vi "poly_average_ith_value_double.vi"(1 "0 indexed? (T, F = 1 indexed)":bool=TRUE, 2 "new value":dbl format="%#_13g", 3 "old value":dbl=nan format="%#_13g", 4 "i":i32) -> (7 "average":dbl)   [LabVIEW 2015]
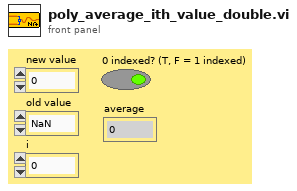
[diagram p1: front panel]
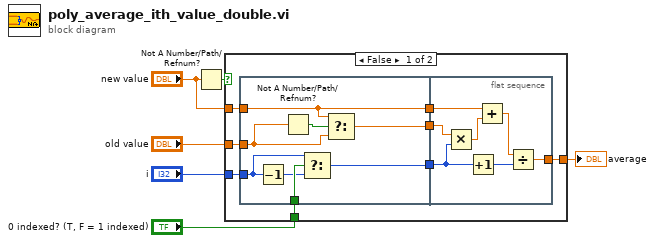
[diagram p0: block diagram]
diagram:
  n1 = Not A Number/Path/Refnum?(number/path/refnum="new value") -> (NaN/Path/Refnum?=w1:bool)
  n2 = case shown="False" w1 {
    tunnel: "old value" -> [w11 w30]
    tunnel: "i" -> [w10 _]
    tunnel: "0 indexed? (T, F = 1 indexed)" -> [w9 _]
    tunnel: [w8 w30] -> w3
    tunnel: "new value" -> [w7 _]
    frame False {
      n3 = flat-sequence {
        tunnel: w11 -> [w17]
        tunnel: w7 -> [w15]
        tunnel: [w16] -> w14
        tunnel: [w21] -> w13
        tunnel: w10 -> [w19]
        tunnel: w9 -> [w20]
        tunnel: [w15] -> w12
        tunnel: w14 -> [w26]
        tunnel: w13 -> [w25]
        tunnel: w12 -> [w24]
        tunnel: [w23] -> w8
        frame #0 {
          n4 = Decrement(x=w19) -> (x-1=w18:i32)
          n5 = Not A Number/Path/Refnum?(number/path/refnum=w17) -> (NaN/Path/Refnum?=w22:bool)
          n6 = Select(t=w19, s=w20, f=w18) -> (s? t:f=w21:i32)
          n7 = Select(t=w15, s=w22, f=w17) -> (s? t:f=w16:dbl)
        }
        frame #1 {
          n8 = Multiply(x=w26, y=w25) -> (x*y=w27:dbl)
          n9 = Increment(x=w25) -> (x+1=w29:i32)
          n10 = Add(x=w24, y=w27) -> (x+y=w28:dbl)
          n11 = Divide(x=w28, y=w29) -> (x/y=w23:dbl)
        }
      }
    }
    frame True {
      # "Do not average the new value if its a NaN"
    }
  }
  "average" <- w3
